vi "NOTIFIER TESTING.vi"() -> ()   [LabVIEW 2017]
panel:
  out "error out 3":errorcluster
  out "error out 2":errorcluster
  out "error out":errorcluster
  out "Numeric 4":i32
  out "Numeric 3":i32
  out "Numeric 2":i32
  out "latest notification 2":dbl
  out "latest notification":dbl
  in  "Numeric":dbl
  out "# waiting 2":i32
  out "# waiting":i32
  in  "Boolean":bool
  in  "stop 3":bool
  in  "stop 2":bool
  in  "stop":bool
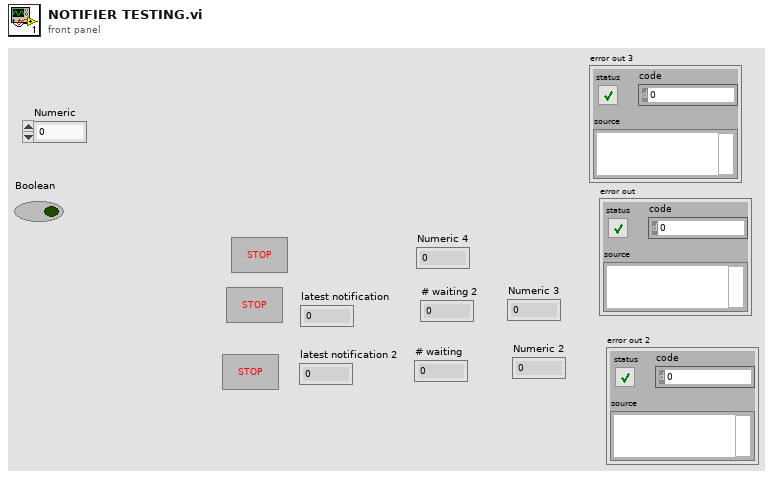
[diagram p1: front panel]
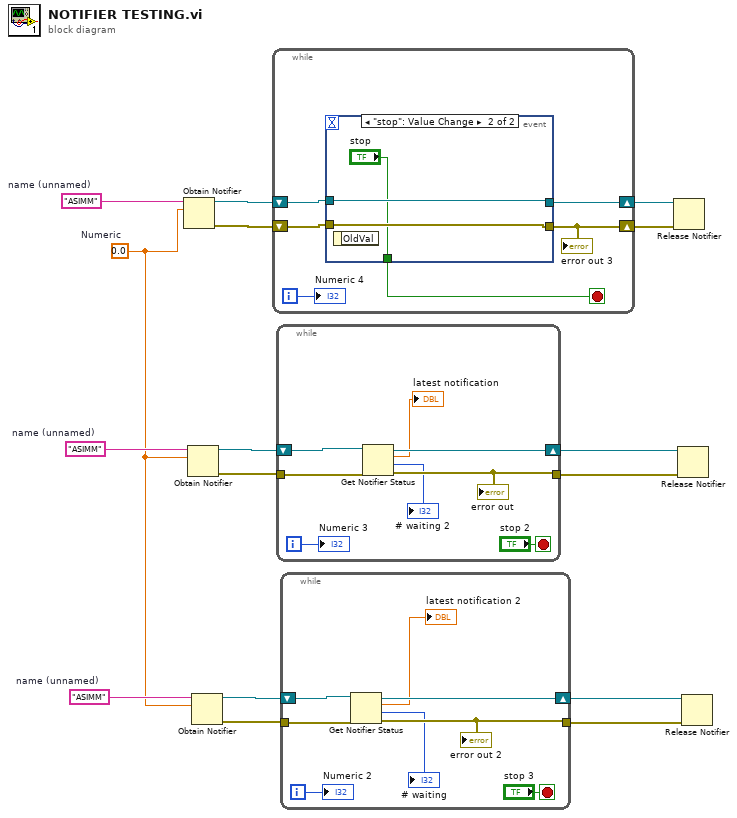
[diagram p0: block diagram]
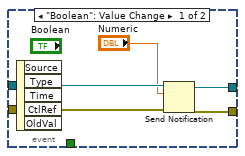
[diagram p2: hidden frame]
diagram:
  w1 = 0.0  # Numeric
  w6 = "ASIMM"  # name (unnamed)
  w7 = "ASIMM"  # name (unnamed)
  w16 = "ASIMM"  # name (unnamed)
  n1 = Obtain Notifier(name (unnamed)=w16, notification data type=w1) -> (notifier out=w15:refnum<notifier>, error out=w14:errorcluster)  [unwired: 2 in, 1 out]
  n2 = Obtain Notifier(name (unnamed)=w7, notification data type=w1) -> (notifier out=w8:refnum<notifier>, error out=w9:errorcluster)  [unwired: 2 in, 1 out]
  n3 = Obtain Notifier(name (unnamed)=w6, notification data type=w1) -> (notifier out=w5:refnum<notifier>, error out=w4:errorcluster)  [unwired: 2 in, 1 out]
  n4 = while {
    shift-right: [w20] -> w13
    shift-left: w15 -> [w22]
    shift-right: [w19] -> w12
    shift-left: w14 -> [w21]
    i -> [w18]
    stop <- w17 stop-if-true
    n5 = event shown="[1] \"stop\": Value Change" {
      selector: _ -> [_ _]
      dyn-events: _ -> [_ _]
      timeout: _ -> [_ _]
      tunnel: w22 -> [w27 w29]
      tunnel: w21 -> [w26 w30]
      tunnel: [w25 w29] -> w20
      tunnel: [w24 w30] -> w19
      tunnel: [_ "stop"] -> w17
      event "Boolean": Value Change {
        n6 = event-data() -> ()  [unwired: 1 in, 5 out]
        n7 = Send Notification(notification="Numeric", notifier=w27, error in (no error)=w26) -> (notifier out=w25:refnum<notifier>, error out=w24:errorcluster)
      }
      event "stop": Value Change {
        n8 = event-data() -> ()  [unwired: 1 in, 1 out]
      }
    }
    "error out 3" <- w19
    "Numeric 4" <- w18
  }
  n9 = while {
    shift-right: [w36] -> w10
    shift-left: w8 -> [w38]
    tunnel: w9 -> [w37]
    tunnel: [w35] -> w11
    i -> [w31]
    stop <- "stop 2" stop-if-true
    n10 = Get Notifier Status(notifier=w38, error in (no error)=w37) -> (notifier out=w36:refnum<notifier>, current notification=→"latest notification":dbl, # waiting=→"# waiting 2":i32, error out=w35:errorcluster)  [unwired: 1 out]
    "error out" <- w35
    "Numeric 3" <- w31
  }
  n11 = while {
    shift-right: [w44] -> w3
    shift-left: w5 -> [w46]
    tunnel: w4 -> [w45]
    tunnel: [w43] -> w2
    i -> [w39]
    stop <- "stop 3" stop-if-true
    n12 = Get Notifier Status(notifier=w46, error in (no error)=w45) -> (notifier out=w44:refnum<notifier>, current notification=→"latest notification 2":dbl, # waiting=→"# waiting":i32, error out=w43:errorcluster)  [unwired: 1 out]
    "error out 2" <- w43
    "Numeric 2" <- w39
  }
  n13 = Release Notifier(notifier=w13, error in (no error)=w12) -> ()  [unwired: 1 in, 3 out]
  n14 = Release Notifier(notifier=w10, error in (no error)=w11) -> ()  [unwired: 1 in, 3 out]
  n15 = Release Notifier(notifier=w3, error in (no error)=w2) -> ()  [unwired: 1 in, 3 out]
